vi "Compute Synchronization Confidence.vi"(0 "Counts for all offsets":u16[][](array[numeric]), 1 "Number of measurements":u16=100, 2 "Confidence (%)":dbl, 5 "Counts for mode offset":u16[](array[numeric]), 11 "error in":errorcluster) -> (4 "Measurements histogram":T1(graph), 15 "error out":errorcluster)   [LabVIEW 2012, in "ni579x Synchronization v1 Host.lvlib"]
uses:
  <instrlib>/ni579x/Synchronization/v1/Host/ni579x Synchronization v1 Host.lvlib
  <vilib>/ErrorRing/Error Ring.xnode
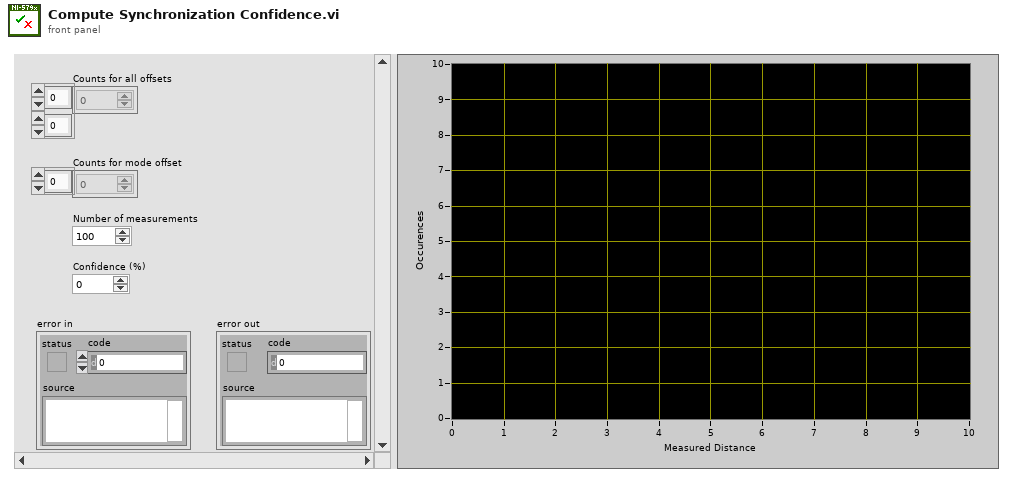
[diagram p1: front panel]
types:
  T1 = cluster{i32[], "Count of offsets (in sample clocks)":u16[]}[]
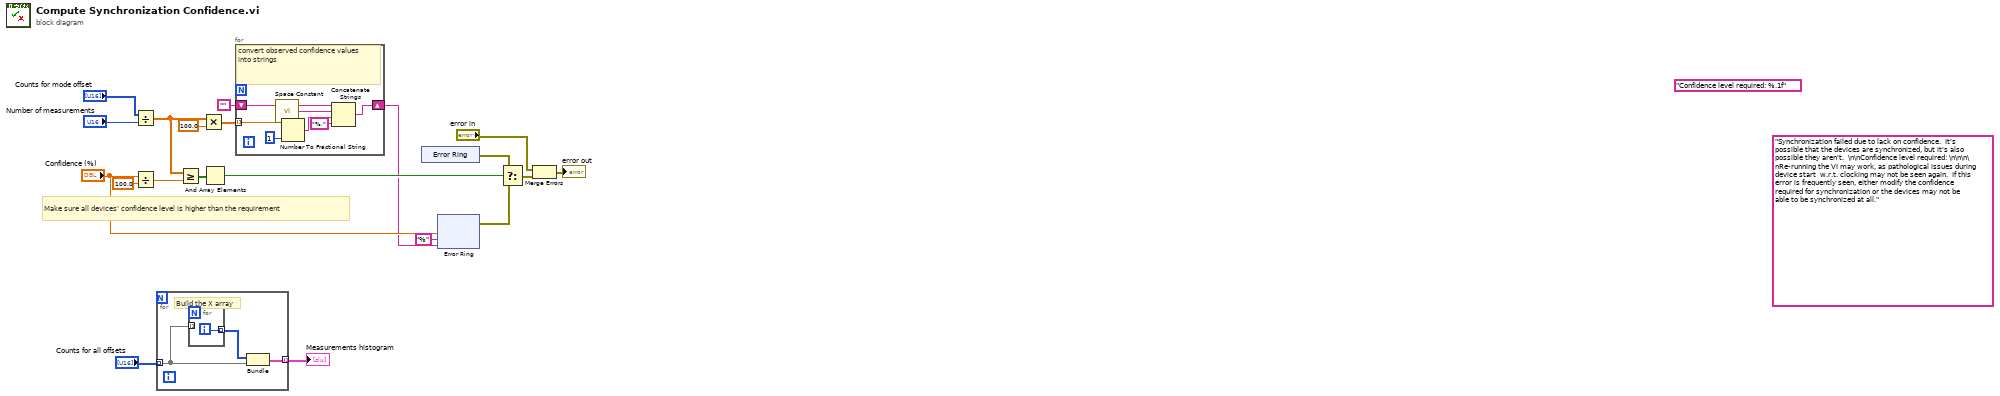
[diagram p0: block diagram]
diagram:
  (unwired) "Synchronization failed due to lack on confidence.  It's possible that the devices are synchronized, but it's also possible they aren't.  \n\nConfidence level required: \n\n\n\nRe-running the VI may work, as pathological issues during device start  w.r.t. clocking may not be seen again.  If this error is frequently seen, either modify the confidence required for synchronization or the devices may not be able to be synchronized at all." ("source")
  (unwired) "Confidence level required: %.1f" ("source")
  # "Make sure all devices' confidence level is higher than the requirement"
  n1 = Divide(x="Counts for mode offset", y="Number of measurements") -> (x/y=w12:dbl[])
  n2 = Divide(x="Confidence (%)", y=100.0) -> (x/y=w14:dbl)
  n3 = for {
    tunnel: "Counts for all offsets" -> [w22] mode=indexing
    tunnel: [w21] -> w9 mode=indexing
    # "Build the X array"
    n4 = for {
      tunnel: w22 -> [_] mode=indexing
      tunnel: [w24] -> w23 mode=indexing
      i -> [w24]
    }
    n5 = Bundle(w23, "Counts for all offsets"=w22) -> (w21:cluster{i32[], "Counts for all offsets":u16[]})  [unwired: 1 in]
  }
  "Measurements histogram" <- w9
  n6 = Greater Or Equal?(x=w12, y=w14) -> (x >= y?=w18:bool[])
  n7 = Multiply(x=w12, y=100.0) -> (x*y=w11:dbl[])
  n8 = And Array Elements(Boolean array=w18) -> (logical AND=w6:bool)
  n9 = for {
    tunnel: w11 -> [w31] mode=indexing
    shift-right: [w25] -> w1
    shift-left: "" -> [w29]
    # "convert observed confidence values into strings"
    n10 = call <vilib>:"Space Constant.vi"() -> ("String"=w28:string)
    n11 = Number To Fractional String(number=w31, precision (6)=i16 1) -> (F-format string=w27:string)  [unwired: 2 in]
    n12 = Concatenate Strings(w29, w28, w27, "%," ("string")) -> (w25:string)
  }
  n13 = xnode "Error Ring"() -> ("error out"=w5:errorcluster)
  n14 = xnode "Error Ring"("parameter 0"="Confidence (%)", "parameter 1"="%", "parameter 2"=w1) -> ("error out"=w4:errorcluster)
  n15 = Select(t=w5, s=w6, f=w4) -> (s? t:f=w3:errorcluster)
  n16 = Merge Errors("error in", w3) -> (→"error out":errorcluster)
